vi "Generate_WayPoints_WITHPAUSE_LED.vi"(4 "Update Position Loop Wait Time (us)":u32=50000, 8 "Feedback Enum":u16=4, 11 "Input Cluster 2":T1={"Scan Rate (um/s)"=15.0, "X Start"=15.0, "X End"=15.0, "Y Start"=15.0, "Y End"=15.0, " Z Start"=15.0, "Number of Lines"=15, "V"=15.0, "Scan Type"=0, "Z End"=15.0, "Approach Rate (um/s)"=15.0, "Squish Approach Rate (um/s)"=15.0, "V 2"=15.0, "HoldTime / us"=15, "Set X"=FALSE, "Set X 2"=FALSE} {"Scan Type" items=["Line Scan (X Major)", "Line Scan (Y Major)"]}) -> (0 "output cluster":T2)   [LabVIEW 2023]
uses:
  TypeDefs/WayPointCluster.ctl
panel:
  in  "WayPointCluster":T2
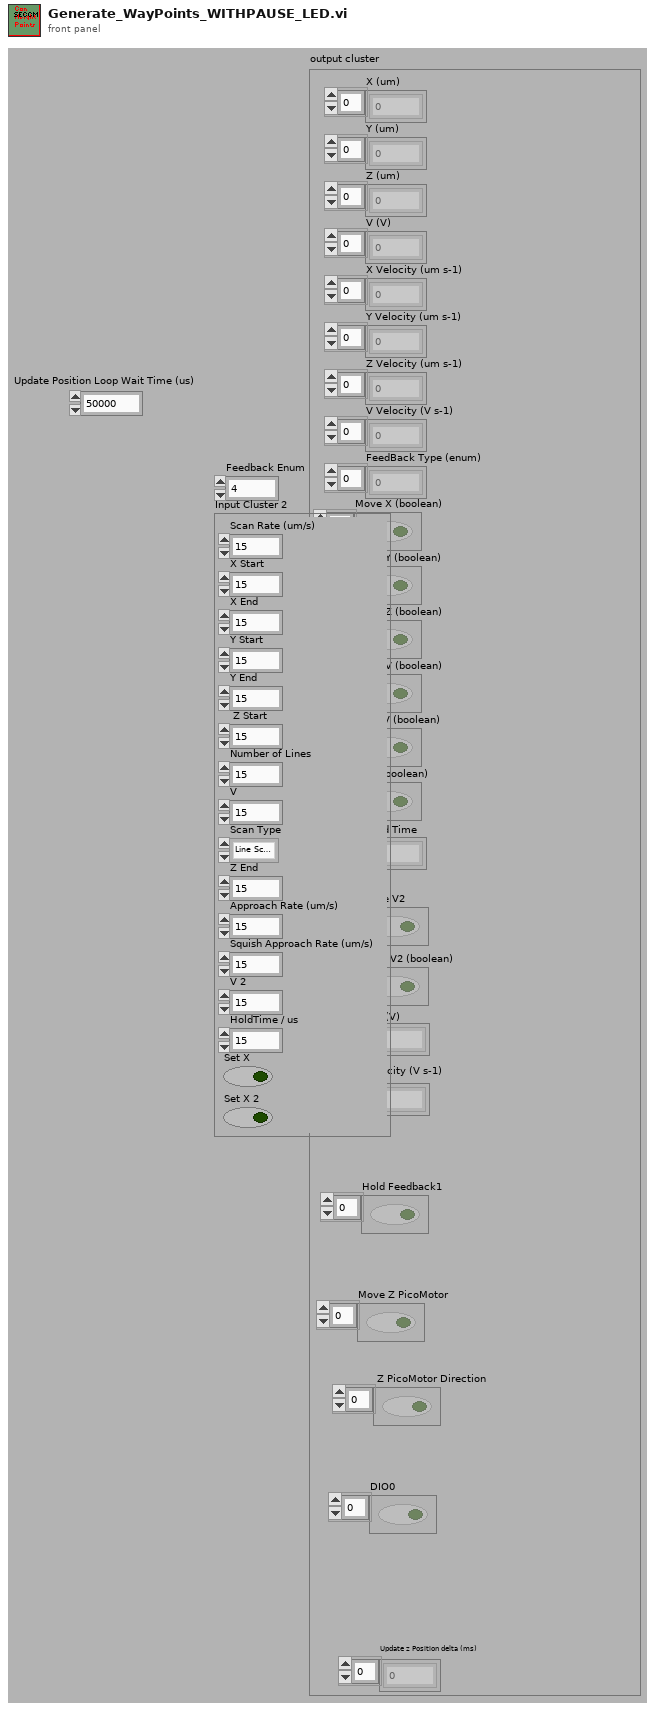
[diagram p1: front panel]
types:
  T1 = cluster{"Scan Rate (um/s)":dbl, "X Start":dbl, "X End":dbl, "Y Start":dbl, "Y End":dbl, " Z Start":dbl, "Number of Lines":u32, "V":dbl, "Scan Type":u16, "Z End":dbl, "Approach Rate (um/s)":dbl, "Squish Approach Rate (um/s)":dbl, "V 2":dbl, "HoldTime / us":u32, "Set X":bool, "Set X 2":bool}
  T2 = typedef "WayPointCluster.ctl" = cluster{"X (um)":dbl[], "Y (um)":dbl[], "Z (um)":dbl[], "V (V)":dbl[], "X Velocity (um s-1)":dbl[], "Y Velocity (um s-1)":dbl[], "Z Velocity (um s-1)":dbl[], "V Velocity (V s-1)":dbl[], "FeedBack Type (enum)":u16[], "Move X (boolean)":bool[], "Move Y (boolean)":bool[], "Move Z (boolean)":bool[], "Move V (boolean)":bool[], "Jump V (boolean)":bool[], "Hold (boolean)":bool[], "Hold Time":u32[], "V2 (V)":dbl[], "Move V2":bool[], "V2 Velocity (V s-1)":dbl[], "Jump V2 (boolean)":bool[], "Update z Position delta (ms)":i16[], "Hold Feedback1":bool[], "Move Z PicoMotor":bool[], " Z PicoMotor Direction":bool[], "DIO0":bool[]}
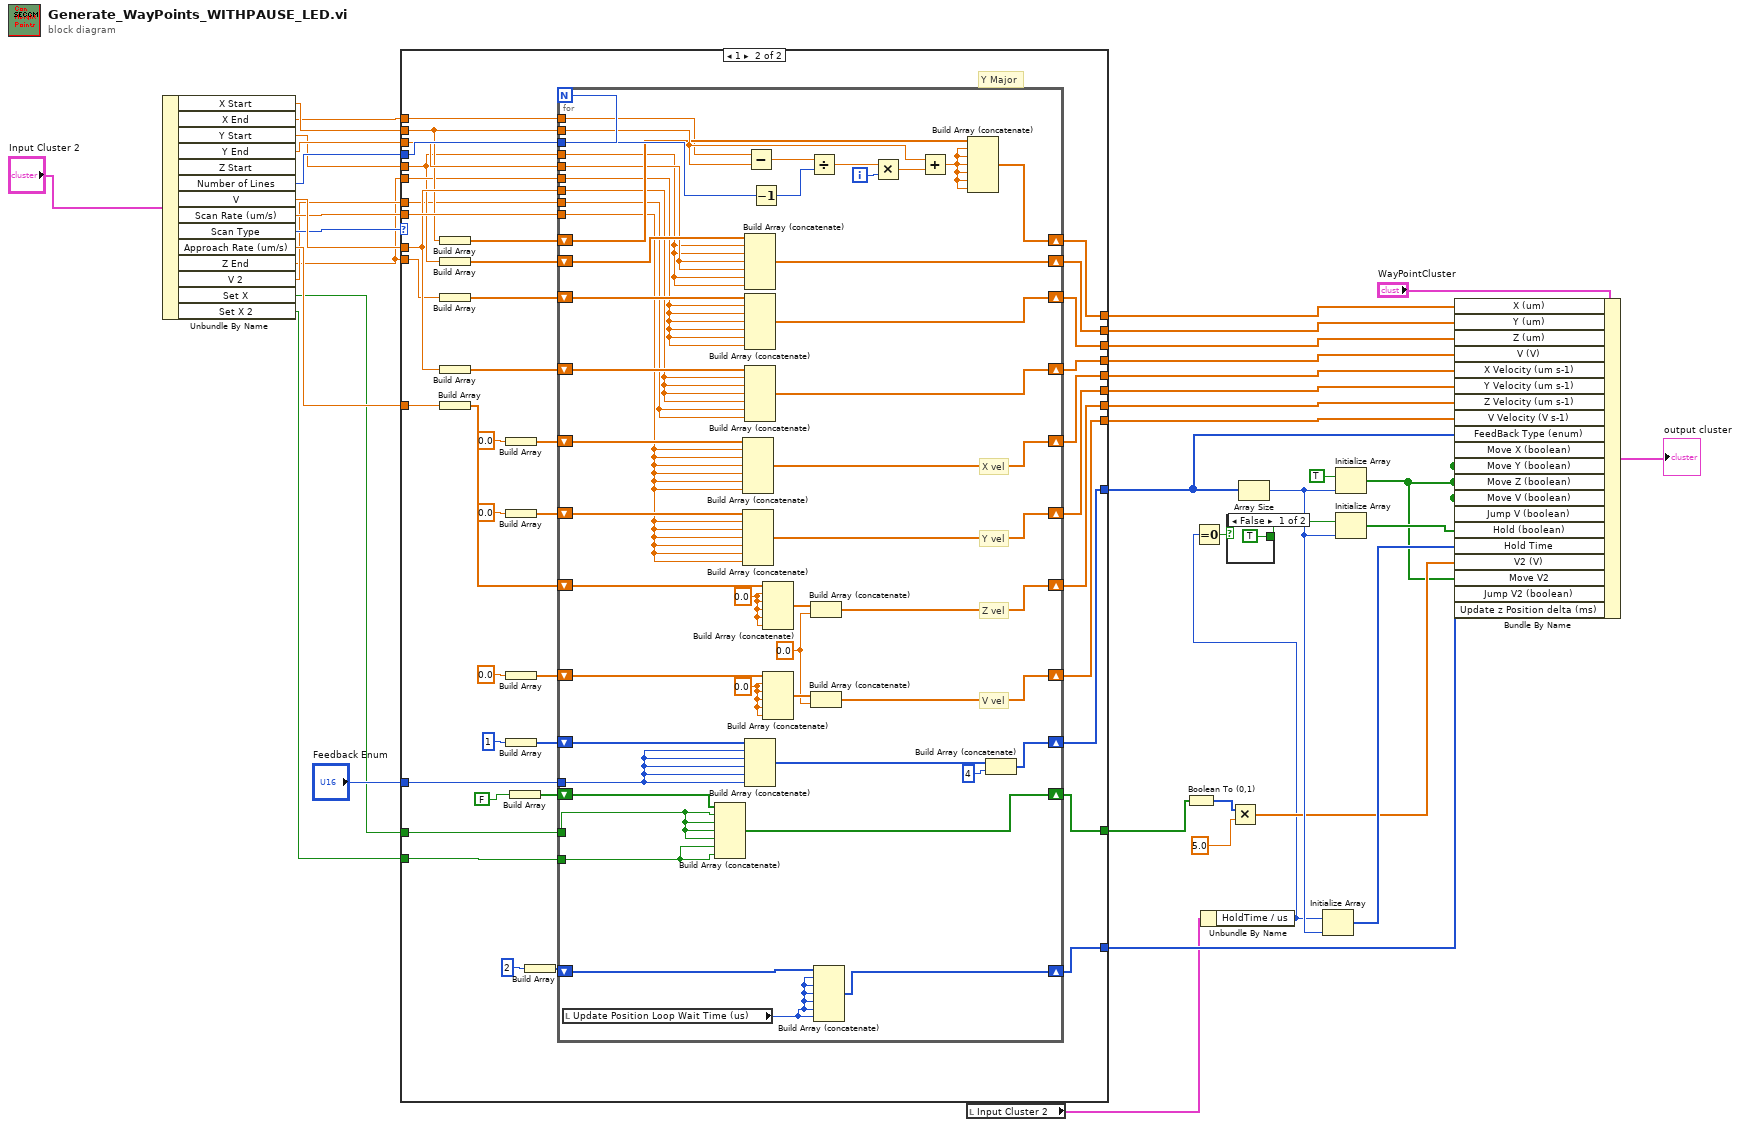
[diagram p0: block diagram]
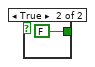
[diagram p2: hidden frame]
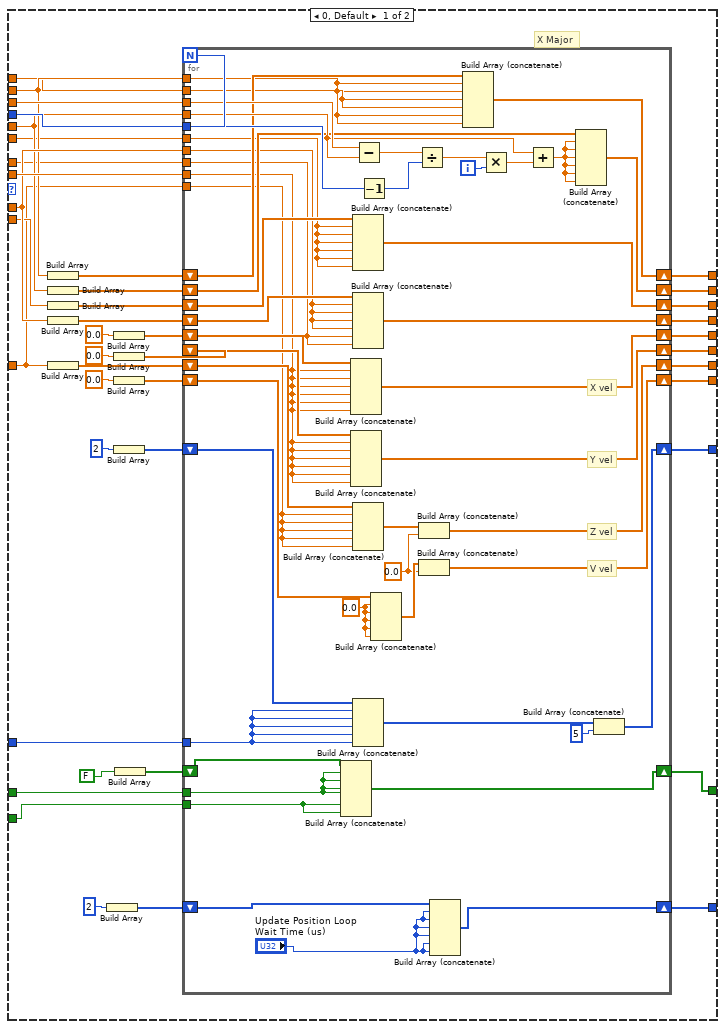
[diagram p3: hidden frame]
diagram:
  n1 = Unbundle By Name("Input Cluster 2") -> ("X Start"=w39:dbl, "X End"=w26:dbl, "Y Start"=w25:dbl, "Y End"=w36:dbl, "Number of Lines"=w38:u32, "V"=w40:dbl, "Scan Rate (um/s)"=w37:dbl, "Scan Type"=w30:u16, "Approach Rate (um/s)"=w27:dbl, "Z End"=w18:dbl, "V 2"=w22:dbl, "Set X"=w11:bool, "Set X 2"=w12:bool)  [unwired: 1 out]
  n2 = case shown="1" w30 {
    tunnel: w40 -> [w62 w149]
    tunnel: w39 -> [w55 w145]
    tunnel: w18 -> [w54 w147]
    tunnel: w38 -> [w82 w172]
    tunnel: w37 -> [w81 w167]
    tunnel: w25 -> [w58 w141]
    tunnel: w36 -> [w80 w164]
    tunnel: [w79 w162] -> w35
    tunnel: [w78 w165] -> w29
    tunnel: [w77 w171] -> w28
    tunnel: [w76 w166] -> w34
    tunnel: [w75 w170] -> w10
    tunnel: [w74 w163] -> w33
    tunnel: [w73 w169] -> w32
    tunnel: [w72 w168] -> w31
    tunnel: w27 -> [w50 w155]
    tunnel: [w71 w161] -> w23
    tunnel: w18 -> [w53 w144]
    tunnel: w26 -> [w52 w143]
    tunnel: w22 -> [w51 w140]
    tunnel: "Feedback Enum" -> [w49 w139]
    tunnel: w12 -> [w45 w136]
    tunnel: w11 -> [w46 w137]
    tunnel: [w44 w134] -> w7
    tunnel: [w41 w131] -> w5
    frame 0, Default {
      # "X Major"
      n3 = Build Array(w55) -> (w56:dbl[])
      n4 = Build Array(w58) -> (w57:dbl[])
      n5 = Build Array(w54) -> (w59:dbl[])
      n6 = Build Array(w62) -> (w61:dbl[])
      n7 = Build Array(w50) -> (w66:dbl[])
      n8 = Build Array(u16 2 ("element")) -> (w43:u16[])
      n9 = Build Array(0.0 ("element")) -> (w63:dbl[])
      n10 = Build Array(0.0 ("element")) -> (w64:dbl[])
      n11 = Build Array(0.0 ("element")) -> (w67:dbl[])
      n12 = Build Array(u16 2 ("element")) -> (w69:u16[])
      n13 = Build Array(FALSE ("Set X 2")) -> (w47:bool[])
      n14 = for {
        N: w82 -> [_]
        tunnel: w55 -> [w103]
        tunnel: w52 -> [w104]
        tunnel: w53 -> [w100]
        tunnel: w62 -> [w99]
        tunnel: w58 -> [w129]
        tunnel: w80 -> [w130]
        tunnel: w82 -> [w125]
        tunnel: w81 -> [w92]
        shift-right: [w94] -> w79
        shift-left: w63 -> [w124]
        shift-right: [w115] -> w78
        shift-left: w57 -> [w123]
        shift-right: [w113] -> w77
        shift-left: w61 -> [w105]
        shift-right: [w116] -> w76
        shift-left: w56 -> [w122]
        shift-right: [w114] -> w75
        shift-left: w59 -> [w121]
        shift-right: [w93] -> w74
        shift-left: w64 -> [w120]
        shift-right: [w109] -> w72
        shift-left: w66 -> [w119]
        shift-right: [w110] -> w73
        shift-left: w67 -> [w118]
        shift-right: [w106] -> w71
        shift-left: w69 -> [w108]
        tunnel: w51 -> [w98]
        tunnel: w50 -> [w91]
        tunnel: w49 -> [w90]
        shift-right: [w86] -> w44
        shift-left: w47 -> [w89]
        tunnel: w46 -> [w88]
        tunnel: w45 -> [w87]
        shift-right: [w83] -> w41
        shift-left: w43 -> [w85]
        i -> [w101]
        w96 = 0.0 ("element")
        w97 = 0.0 ("element")
        # "Y vel"
        # "X vel"
        # "Z vel"
        # "V vel"
        n15 = Build Array (concatenate)(w89, w88, w88, w88, w88, w87, w87) -> (w86:bool[])
        n16 = Build Array (concatenate)(w124, w92, w92, w92, w92, w92, w92) -> (w94:dbl[])
        n17 = Build Array (concatenate)(w120, w92, w92, w92, w92, w92, w92) -> (w93:dbl[])
        n18 = Build Array (concatenate)(w121, w100, w100, w100, w100, w100, w100) -> (w114:dbl[])
        n19 = Build Array (concatenate)(w105, w99, w99, w99, w99, w98, w98) -> (w113:dbl[])
        n20 = Build Array (concatenate)(w119, w91, w91, w91, w91, w91) -> (w112:dbl[])
        n21 = Build Array (concatenate)(w108, w90, w90, w90, w90, w90) -> (w107:u16[])
        n22 = Subtract(x=w130, y=w129) -> (x-y=w128:dbl)
        n23 = Decrement(x=w125) -> (x-1=w117:u32)
        n24 = Build Array (concatenate)(w118, w97, w97, w97, w97, w97) -> (w111:dbl[])
        n25 = Divide(x=w128, y=w117) -> (x/y=w126:dbl)
        n26 = Build Array (concatenate)(w112, w96) -> (w109:dbl[])
        n27 = Build Array (concatenate)(w111, w96) -> (w110:dbl[])
        n28 = Build Array (concatenate)(w85, "Update Position Loop Wait Time (us)", "Update Position Loop Wait Time (us)", "Update Position Loop Wait Time (us)", "Update Position Loop Wait Time (us)", "Update Position Loop Wait Time (us)", "Update Position Loop Wait Time (us)") -> (w83:u32[])
        n29 = Build Array (concatenate)(w122, w103, w103, w104, w104, w103, w103) -> (w116:dbl[])
        n30 = Multiply(x=w126, y=w101) -> (x*y=w127:dbl)
        n31 = Add(x=w129, y=w127) -> (x+y=w102:dbl)
        n32 = Build Array (concatenate)(w123, w102, w102, w102, w102, w102, w102) -> (w115:dbl[])
        n33 = Build Array (concatenate)(w107, u16 5 ("element")) -> (w106:u16[])
      }
    }
    frame 1 {
      # "Y Major"
      n34 = Build Array(w145) -> (w146:dbl[])
      n35 = Build Array(w141) -> (w142:dbl[])
      n36 = Build Array(w147) -> (w148:dbl[])
      n37 = Build Array(w149) -> (w150:dbl[])
      n38 = Build Array(w155) -> (w156:dbl[])
      n39 = Build Array(0.0 ("element")) -> (w151:dbl[])
      n40 = Build Array(0.0 ("element")) -> (w153:dbl[])
      n41 = Build Array(0.0 ("element")) -> (w159:dbl[])
      n42 = Build Array(u16 1 ("element")) -> (w157:u16[])
      n43 = Build Array(FALSE ("Set X 2")) -> (w135:bool[])
      n44 = Build Array(u16 2 ("element")) -> (w132:u16[])
      n45 = for {
        N: w172 -> [_]
        tunnel: w141 -> [w192]
        tunnel: w164 -> [w193]
        tunnel: w144 -> [w191]
        tunnel: w149 -> [w190]
        tunnel: w145 -> [w220]
        tunnel: w172 -> [w216]
        tunnel: w167 -> [w181]
        shift-right: [w183] -> w162
        shift-left: w151 -> [w205]
        shift-right: [w202] -> w166
        shift-left: w146 -> [w215]
        shift-right: [w199] -> w171
        shift-left: w150 -> [w214]
        shift-right: [w201] -> w165
        shift-left: w142 -> [w213]
        shift-right: [w200] -> w170
        shift-left: w148 -> [w212]
        shift-right: [w182] -> w163
        shift-left: w153 -> [w204]
        shift-right: [w208] -> w168
        shift-left: w156 -> [w211]
        shift-right: [w209] -> w169
        shift-left: w159 -> [w210]
        shift-right: [w195] -> w161
        shift-left: w157 -> [w197]
        tunnel: w143 -> [w194]
        tunnel: w140 -> [w189]
        tunnel: w139 -> [w180]
        tunnel: w137 -> [w178]
        tunnel: w136 -> [w177]
        shift-right: [w176] -> w134
        shift-left: w135 -> [w179]
        shift-right: [w173] -> w131
        shift-left: w132 -> [w175]
        i -> [w207]
        w185 = 0.0 ("element")
        w187 = 0.0 ("element")
        w186 = 0.0 ("element")
        # "Y vel"
        # "X vel"
        # "Z vel"
        # "V vel"
        n46 = local read "Update Position Loop Wait Time (us)"() -> (w174:u32)
        n47 = Build Array (concatenate)(w179, w178, w178, w178, w178, w177, w177) -> (w176:bool[])
        n48 = Build Array (concatenate)(w205, w181, w181, w181, w181, w181, w181) -> (w183:dbl[])
        n49 = Build Array (concatenate)(w204, w181, w181, w181, w181, w181, w181) -> (w182:dbl[])
        n50 = Build Array (concatenate)(w213, w192, w192, w193, w193, w192, w192) -> (w201:dbl[])
        n51 = Build Array (concatenate)(w212, w191, w191, w191, w191, w191, w191) -> (w200:dbl[])
        n52 = Build Array (concatenate)(w214, w190, w190, w190, w190, w189, w189) -> (w199:dbl[])
        n53 = Build Array (concatenate)(w197, w180, w180, w180, w180, w180) -> (w196:u16[])
        n54 = Subtract(x=w194, y=w220) -> (x-y=w219:dbl)
        n55 = Decrement(x=w216) -> (x-1=w206:u32)
        n56 = Build Array (concatenate)(w211, w186, w186, w186, w186, w186) -> (w198:dbl[])
        n57 = Build Array (concatenate)(w210, w187, w187, w187, w187, w187) -> (w203:dbl[])
        n58 = Divide(x=w219, y=w206) -> (x/y=w217:dbl)
        n59 = Build Array (concatenate)(w198, w185) -> (w208:dbl[])
        n60 = Build Array (concatenate)(w203, w185) -> (w209:dbl[])
        n61 = Build Array (concatenate)(w175, w174, w174, w174, w174, w174, w174) -> (w173:u32[])
        n62 = Multiply(x=w217, y=w207) -> (x*y=w218:dbl)
        n63 = Add(x=w220, y=w218) -> (x+y=w188:dbl)
        n64 = Build Array (concatenate)(w215, w188, w188, w188, w188, w188, w188) -> (w202:dbl[])
        n65 = Build Array (concatenate)(w196, u16 4 ("element")) -> (w195:u16[])
      }
    }
  }
  n66 = local read "Input Cluster 2"() -> (w1:T1)
  n67 = Boolean To (0,1)(Boolean=w7) -> (0, 1=w9:i16[])
  n68 = Unbundle By Name(w1) -> ("HoldTime / us"=w2:u32)
  n69 = Equal To 0?(x=w2) -> (x = 0?=w3:bool)
  n70 = case shown="False" w3 {
    tunnel: [TRUE FALSE] -> w21
    frame False {
    }
    frame True {
    }
  }
  n71 = Multiply(x=w9, y=5.0) -> (x*y=w6:dbl[])
  n72 = Array Size(array=w23) -> (size(s)=w20:i32)
  n73 = Initialize Array(w2, w20) -> (w19:u32[])
  n74 = Initialize Array(TRUE, w20) -> (w4:bool[])
  n75 = Initialize Array(w21, w20) -> (w13:bool[])
  n76 = Bundle By Name(cluster="WayPointCluster", "X (um)"=w34, "Y (um)"=w29, "Z (um)"=w10, "V (V)"=w28, "X Velocity (um s-1)"=w35, "Y Velocity (um s-1)"=w33, "Z Velocity (um s-1)"=w31, "V Velocity (V s-1)"=w32, "FeedBack Type (enum)"=w23, "Move X (boolean)"=w4, "Move Y (boolean)"=w4, "Move Z (boolean)"=w4, "Move V (boolean)"=w4, "Jump V (boolean)"=w4, "Hold (boolean)"=w13, "Hold Time"=w19, "V2 (V)"=w6, "Move V2"=w4, "Jump V2 (boolean)"=w4, "Update z Position delta (ms)"=w5) -> (→"output cluster":T2)
